vi "FPGA_acquisition - 9205.vi"(8 "error in (no error)":errorcluster, 10 "pound in":refnum<class "Pound.lvclass">, 11 "qbus in":refnum<class "Qbus.lvclass">) -> (0 "error out":errorcluster)   [LabVIEW 2015]
uses:
  <vilib>/addons/Qbus/Qbus.lvclass
  <vilib>/NI/Software Watchdog/Pound/Pound.lvclass
  <vilib>/addons/InsightCM/Devices/Shared/AcquireBaseLoop/controls/State.ctl
  <vilib>/addons/InsightCM/Devices/Shared/AcquireBaseLoop/controls/Configuration.ctl
  <vilib>/addons/InsightCM/Devices/Shared/AcquireBaseLoop/controls/TachometerConfig.ctl
  <vilib>/addons/InsightCM/Devices/Shared/AcquireBaseLoop/controls/FixedSizeArrays.ctl
  <vilib>/LabVIEW Targets/FPGA/cRIO/shared/nicrio_ModuleControls/nicrio_cRIO-9232_ConfigModeRing.ctl
  <vilib>/addons/InsightCM/Devices/Shared/cRIOWfmAcq/subVIs/RIO Wfm Cust Ctrls/rwfm_SamplingInfo.ctl
  <vilib>/addons/InsightCM/Devices/Shared/AcquireBaseLoop/controls/Group.ctl
  <vilib>/addons/InsightCM/Devices/Shared/AcquireBaseLoop/controls/Channel.ctl
  <vilib>/addons/InsightCM/Utilities/ChannelStatus/controls/RangeParams.ctl
  <vilib>/addons/InsightCM/Devices/Shared/AcquireBaseLoop/FpgaAcquisition923x.lvlib
  <vilib>/addons/InsightCM/Devices/Shared/TdmsCreator/TdmsCreator.lvlib
  <vilib>/addons/InsightCM/Devices/Shared/TagPublish/TagPublish.lvlib
  <vilib>/addons/InsightCM/Devices/Shared/FPGABitfileManager/FPGABitfileManager.lvlib
  <vilib>/addons/InsightCM/Devices/Shared/cRIOWfmAcq/cRIOWfmLib.lvlib
  <vilib>/addons/InsightCM/Devices/Shared/DataFlow/DataFlow.lvlib
  <vilib>/addons/InsightCM/Devices/Shared/QbusHelpers/QbusHelper.lvlib
  <vilib>/NI/Software Watchdog/Watchdog/Watchdog.lvclass
  <vilib>/addons/InsightCM/Utilities/ChannelStatus/ChannelStatus.lvlib
panel:
  in  "Waveform Groups Empty?":bool
  out "Numeric":i32
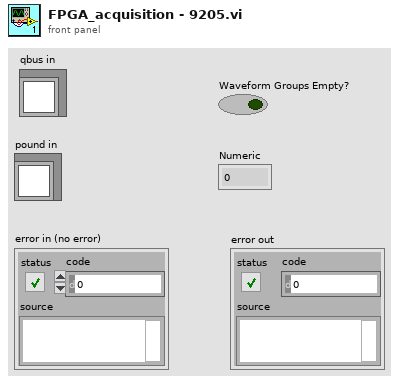
[diagram p1: front panel]
types:
  T1 = typedef "FpgaAcquisition923x.lvlib/Configuration.ctl" = cluster{"NumberOfModules":i16, "Dynamic FPGA VI Ref":refnum<k20>, "KeyphasorX3":T2[], "FixedSizeX24":T3, "SamplingInfo":T5, "BlockSize (sec)":dbl, "Samples To Read (per chan)":i32, "RunningAcquisitionLength":dbl, "Settling Time":dbl, "Waveform Groups":T6[], "Acquisition Block Number":i32, "Device Name":string, "ValidConfig":bool}
  T2 = typedef "FpgaAcquisition923x.lvlib/TachometerConfig.ctl" = cluster{"slope":enum16{"falling", "rising"}, "threshold":dbl, "hysteresis":dbl}
  T3 = typedef "FpgaAcquisition923x.lvlib/FixedSizeArrays.ctl" = cluster{"EnabledChannels":bool[], "Sensitivity":dbl[], "InputConfig":T4[]}
  T4 = typedef "nicrio_cRIO-9232_ConfigModeRing.ctl" = u8
  T5 = typedef "cRIOWfmLib.lvlib/rwfm_SamplingInfo.ctl" = cluster{"Number of Channels":i32, "Sampling Rate":dbl, "Channels":string[], "Units":string[]}
  T6 = typedef "FpgaAcquisition923x.lvlib/Group.ctl" = cluster{"Name":string, "Speed Reference":string, "Channels":T7[]}
  T7 = typedef "FpgaAcquisition923x.lvlib/Channel.ctl" = cluster{"Name":string, "Status Tag":string, "RangeCheck":T8}
  T8 = typedef "ChannelStatus.lvlib/RangeParams.ctl" = cluster{"Enabled":bool, "Max":dbl, "Min":dbl}
  T9 = typedef "FpgaAcquisition923x.lvlib/State.ctl" = enum16{"Unconfigured", "Configured"}
  T10 = typedef "TagPublish.lvlib/PointToPublish.ctl" = cluster{"Id":string, "datatype":T11}
  T11 = typedef "PointValueMap.lvlib/DataTypes.ctl" = enum16{"single", "double", "i32", "string", "variant"}
  T12 = typedef "TdmsCreator.lvlib/RegisterWaveformTdmsPropertiesRoutedMessage.ctl" = cluster{"DataGroup":string, "TdmsGroup":string, "Channels":T13[]}
  T13 = typedef "TdmsCreator.lvlib/Waveform.ctl" = cluster{"ChannelName":string, "Properties":variant, "Write Wfm":bool}
  T14 = typedef "DataFlow.lvlib/Data.ctl" = cluster{"DataGroup":string, "Waveforms":T15, "Map":T16}
  T15 = typedef "wfmSGL_DVR.ctl" = refnum<data-value>
  T16 = typedef "PointValueMap.lvlib/PointMap.ctl" = refnum<data-value>
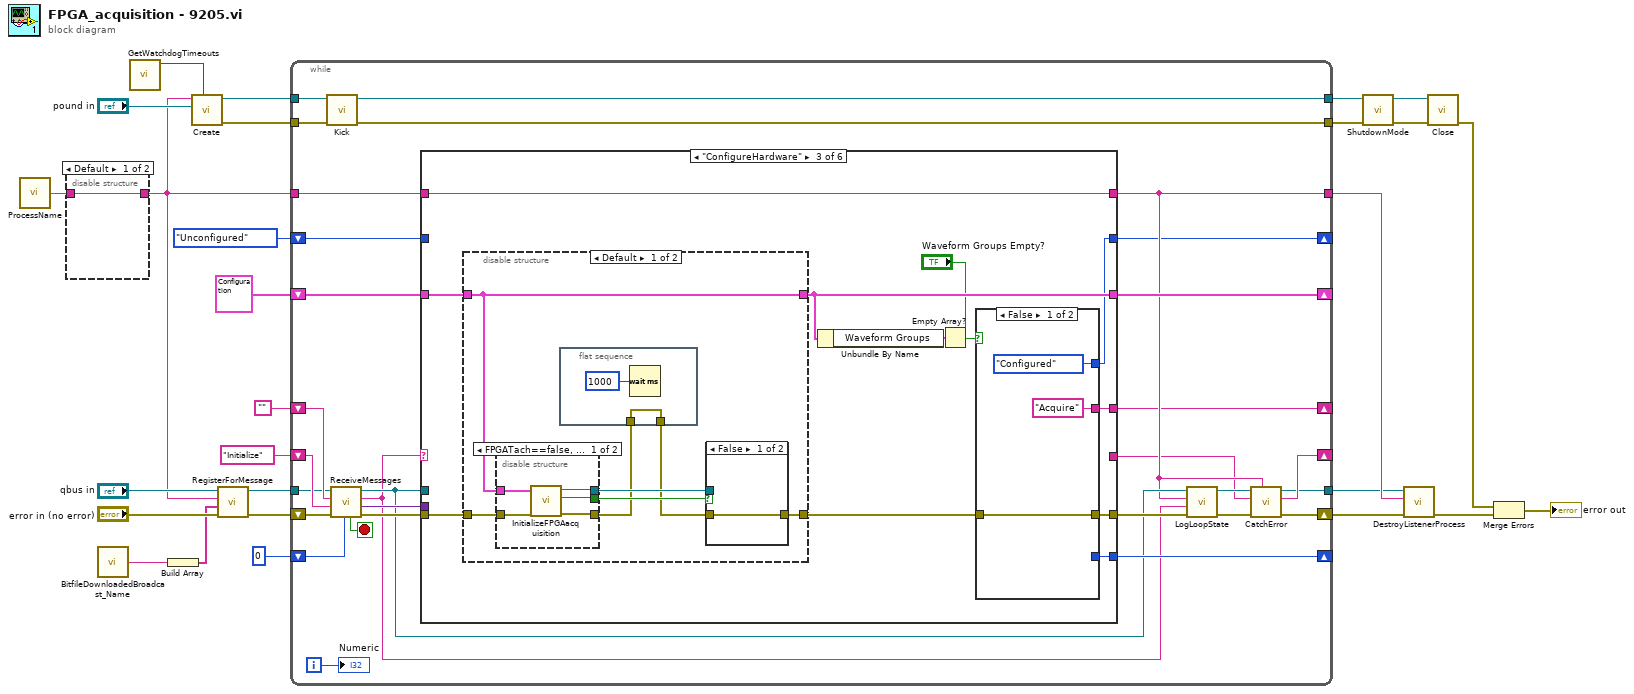
[diagram p0: block diagram]
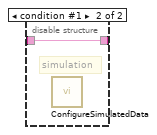
[diagram p2: hidden frame]
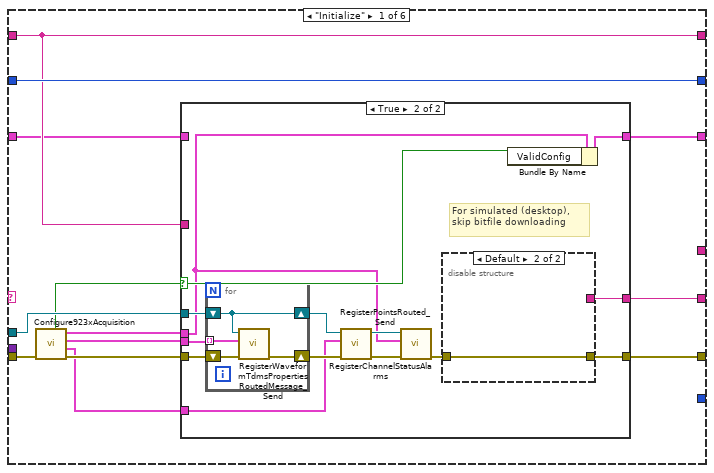
[diagram p3: hidden frame]
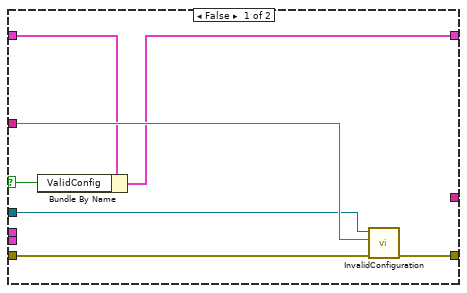
[diagram p4: hidden frame]
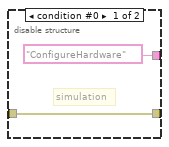
[diagram p5: hidden frame]
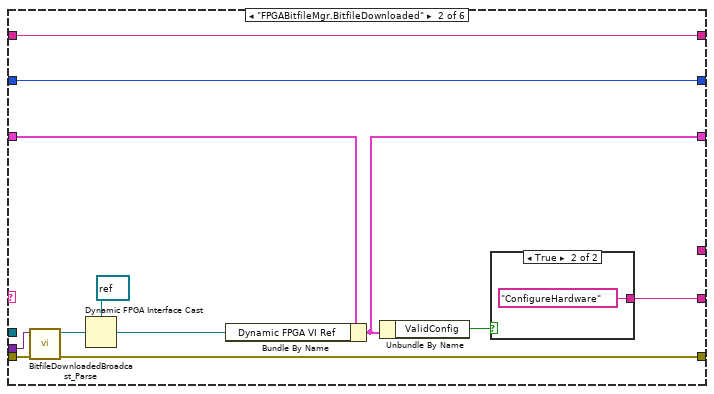
[diagram p6: hidden frame]
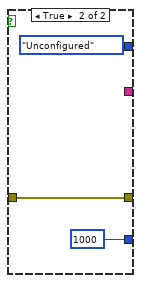
[diagram p8: hidden frame]
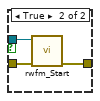
[diagram p9: hidden frame]
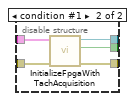
[diagram p10: hidden frame]
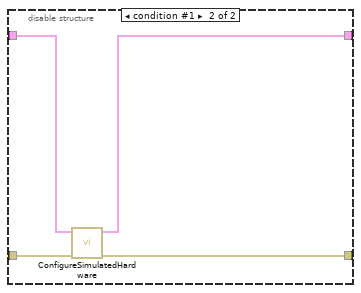
[diagram p11: hidden frame]
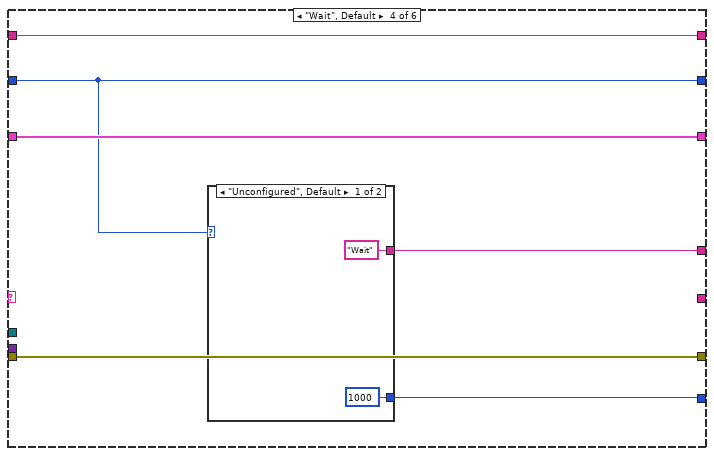
[diagram p12: hidden frame]
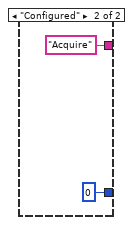
[diagram p13: hidden frame]
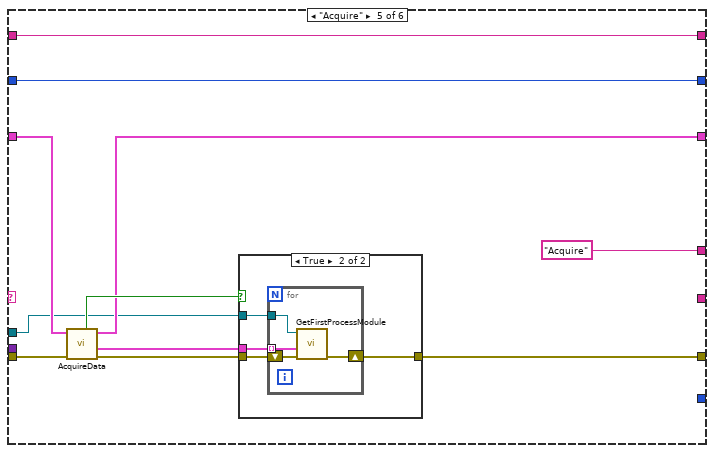
[diagram p14: hidden frame]
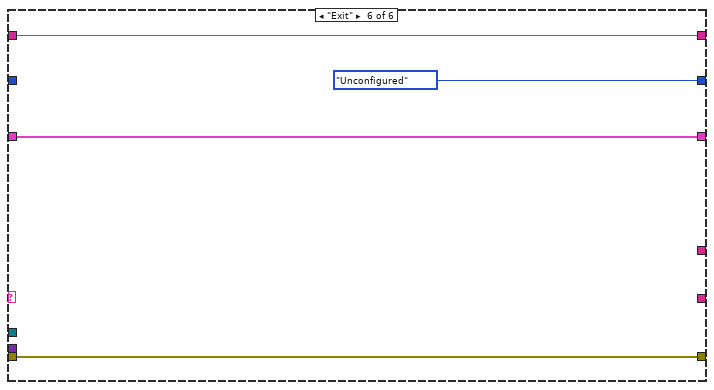
[diagram p16: hidden frame]
diagram:
  n1 = call <vilib>:"ProcessName.vi"() -> ("process name"=w5:string)  [unwired: 5 in]
  n2 = disable-structure shown="Default" {
    disable-tunnel: [w28 w29] -> w6
    disable-tunnel: w5 -> [w28 w29]
    frame condition #0 (active) {
    }
    frame condition #1 {
      # "simulation"
      n3 = call <vilib>:"ConfigureSimulatedData.vi"() -> ()  [unwired: 11 in, 1 out]
    }
  }
  n4 = call <vilib>:"BitfileDownloadedBroadcast_Name.vi"() -> ("message name"=w8:string)  [unwired: 5 in]
  n5 = call <vilib>:"GetWatchdogTimeouts.vi"() -> ("software timeout"=w1:u32)  [unwired: 10 in, 1 out]
  n6 = Build Array(w8) -> (w9:string[])
  n7 = call <vilib>:"Create.vi"("Execution Timeout (ms)"=w1, "Pound"="pound in", "Name"=w6) -> ("error out"=w22:errorcluster, "Watchdog"=w23:refnum<data-value>)  [unwired: 7 in]
  n8 = call <vilib>:"RegisterForMessage.vi"("error in (no error)"="error in (no error)", "message names"=w9, "process name"=w6, "Qbus in"="qbus in") -> ("error in (no error)"=w11:errorcluster, "Qbus out"=w12:refnum<class "Qbus.lvclass">)  [unwired: 6 in]
  n9 = while {
    shift-right: [w46] -> w2
    shift-left: w11 -> [w53]
    shift-right: [w36] -> _
    shift-left: "" -> [w55]
    shift-right: [w59] -> _
    shift-left: T1 {"NumberOfModules"=0, "Dynamic FPGA VI Ref"=refnum, "KeyphasorX3"=[], "FixedSizeX24"={"EnabledChannels"=[], "Sensitivity"=[], "InputConfig"=[]}, "SamplingInfo"={"Number of Channels"=4, "Sampling Rate"=4.0, "Channels"=[], "Units"=[]}, "BlockSize (sec)"=0.0, "Samples To Read (per chan)"=0, "RunningAcquisitionLength"=0.0, "Settling Time"=0.0, "Waveform Groups"=[], "Acquisition Block Number"=0, "Device Name"="", "ValidConfig"=FALSE} ("Config out") -> [w58]
    shift-right: [w34] -> _
    shift-left: State."Unconfigured" ("loop state") -> [w57]
    shift-right: [w56] -> _
    shift-left: 0 ("milliseconds to wait") -> [w51]
    shift-right: [w44] -> _
    shift-left: "Initialize" -> [w54]
    tunnel: w12 -> [w52]
    tunnel: w6 -> [w31]
    tunnel: [w42] -> w3
    tunnel: [w37] -> w25
    tunnel: w23 -> [w41]
    tunnel: w22 -> [w40]
    tunnel: [w39] -> w19
    tunnel: [w38] -> w18
    i -> [w30]
    stop <- w32 stop-if-true
    n10 = call <vilib>:"Kick.vi"("error in (no error)"=w40, "Watchdog"=w41) -> ("error out"=w38:errorcluster, "Watchdog"=w39:refnum<data-value>)  [unwired: 8 in]
    n11 = call <vilib>:"ReceiveMessages.vi"("timeout(100)"=w51, "error in (no error)"=w53, "priority action"=w54, "default action"=w55, "qbus in"=w52) -> ("error out"=w50:errorcluster, "msg value"=w49:variant, "action"=w33:string, "qbus out"=w45:refnum<class "Qbus.lvclass">, "exit"=w32:bool)  [unwired: 2 in]
    n12 = case shown="\"ConfigureHardware\"" w33 {
      tunnel: w50 -> [w70 w104 w122 w163 w170 w188]
      tunnel: [w65 w103 w117 w163 w169 w188] -> w47
      tunnel: [_ _ w124 w161 "Acquire" _] -> w36
      tunnel: [w60 w102 w119 w162 w173 w191] -> w59
      tunnel: w58 -> [w61 w111 w123 w162 w174 w191]
      tunnel: w57 -> [w67 w107 _ w158 w172 _]
      tunnel: [_ _ w116 w159 _ _] -> w56
      tunnel: w31 -> [w63 w112 w121 w160 w171 w189]
      tunnel: w49 -> [_ w105 _ _ _ _]
      tunnel: w45 -> [w69 _ _ _ w168 _]
      tunnel: [w63 w112 w121 w160 w171 w189] -> w37
      tunnel: [w68 w108 _ _ _ _] -> w35
      tunnel: [w67 w107 w115 w158 w172 State."Unconfigured" ("loop state")] -> w34
      frame "Initialize" {
        n13 = call <vilib>:"Configure923xAcquisition.vi"("error in (no error)"=w70) -> ("error out"=w72:errorcluster, "Register Channel Status Tags"=w66:T10[], "Register Waveform TDMS Properties"=w71:T12[], "923x Acquisition Config"=w64:T1, "valid"=w62:bool)  [unwired: 6 in]
        n14 = case shown="True" w62 {
          selector: w62 -> [w75 w81]
          tunnel: w72 -> [w73 w93]
          tunnel: w71 -> [_ w92]
          tunnel: w69 -> [w74 w91]
          tunnel: [_ w90] -> w68
          tunnel: w66 -> [_ w88]
          tunnel: [w79 w83] -> w65
          tunnel: w64 -> [_ w80]
          tunnel: w63 -> [w78 _]
          tunnel: w61 -> [w77 _]
          tunnel: [w76 w82] -> w60
          frame False {
            n15 = Bundle By Name(cluster=w77, "ValidConfig"=w75) -> (w76:T1)
            n16 = call <vilib>:"InvalidConfiguration.vi"("error in (no error)"=w73, "description"=w78, "Qbus in"=w74) -> ("error out"=w79:errorcluster)  [unwired: 7 in, 1 out]
          }
          frame True {
            # "For simulated (desktop),\nskip bitfile downloading"
            n17 = for {
              shift-right: [w99] -> w89
              shift-left: w93 -> [w100]
              tunnel: w92 -> [w98] mode=indexing
              shift-right: [w97] -> w87
              shift-left: w91 -> [w97]
              n18 = call <vilib>:"RegisterWaveformTdmsPropertiesRoutedMessage_Send.vi"("error in (no error)"=w100, "register waveform"=w98, "Qbus in"=w97) -> ("error out"=w99:errorcluster)  [unwired: 7 in, 1 out]
            }
            n19 = call <vilib>:"RegisterPointsRouted_Send.vi"("error in (no error)"=w89, "points"=w88, "Qbus in"=w87) -> ("error out"=w86:errorcluster, "Qbus out"=w84:refnum<class "Qbus.lvclass">)  [unwired: 7 in]
            n20 = call <vilib>:"RegisterChannelStatusAlarms.vi"("error in (no error)"=w86, "923x Acquisition Config"=w80, "Qbus in"=w84) -> ("error out"=w85:errorcluster)  [unwired: 8 in]
            n21 = disable-structure shown="Default" {
              disable-tunnel: w85 -> [w94 w96]
              disable-tunnel: [w94 w96] -> w83
              disable-tunnel: ["ConfigureHardware" _] -> w90
              frame condition #0 {
                # "simulation"
              }
              frame condition #1 (active) {
              }
            }
            n22 = Bundle By Name(cluster=w80, "ValidConfig"=w81) -> (w82:T1)
          }
        }
      }
      frame "FPGABitfileMgr.BitfileDownloaded" {
        n23 = call <vilib>:"BitfileDownloadedBroadcast_Parse.vi"("error in (no error)"=w104, "data"=w105) -> ("error out"=w103:errorcluster, "FPGA reference"=w106:refnum<k20>)  [unwired: 8 in]
        n24 = Dynamic FPGA Interface Cast(Session In=refnum<k20> refnum ("Dynamic FPGA VI Ref"), Type=w106) -> (Session Out=w110:refnum<k20>)
        n25 = Bundle By Name(cluster=w111, "Dynamic FPGA VI Ref"=w110) -> (w102:T1)
        n26 = Unbundle By Name(w102) -> ("ValidConfig"=w101:bool)
        n27 = case shown="True" w101 {
          tunnel: [_ "ConfigureHardware"] -> w108
          frame False {
          }
          frame True {
          }
        }
      }
      frame "ConfigureHardware" {
        n28 = disable-structure shown="Default" {
          disable-tunnel: w123 -> [w134 w155]
          disable-tunnel: w122 -> [w137 w157]
          disable-tunnel: [w136 w156] -> w118
          disable-tunnel: [w134 w154] -> w119
          frame condition #0 (active) {
            n29 = disable-structure shown="FPGATach==false, Default" {
              disable-tunnel: w137 -> [w147 w153]
              disable-tunnel: [w144 w151] -> w132
              disable-tunnel: w134 -> [w148 w152]
              disable-tunnel: [w146 w150] -> w135
              disable-tunnel: [w145 w149] -> w133
              frame condition #0 (active) {
                n30 = call "InitializeFPGAacquisition.vi"("error in (no error)"=w147, "923x Acquisition Config"=w148) -> ("error out"=w144:errorcluster, "start acquisition?"=w145:bool, "dynamic FPGA VI reference"=w146:refnum<k20>)  [unwired: 5 in, 2 out]
              }
              frame condition #1 {
                n31 = call <vilib>:"InitializeFpgaWithTachAcquisition.vi"("error in (no error)"=w153, "923x Acquisition Config"=w152) -> ("error out"=w151:errorcluster, "start acquisition?"=w149:bool, "dynamic FPGA VI reference"=w150:refnum<k20>)  [unwired: 7 in]
              }
            }
            n32 = flat-sequence {
              tunnel: [w138] -> w131
              tunnel: w132 -> [w138]
              frame #0 {
                n33 = Wait (ms)(milliseconds to wait=u32 1000) -> ()  [unwired: 1 out]
              }
            }
            n34 = case shown="False" w133 {
              tunnel: [w140 w143] -> w136
              tunnel: w131 -> [w140 w142]
              tunnel: w135 -> [_ w141]
              frame False {
              }
              frame True {
                n35 = call <vilib>:"rwfm_Start.vi"("error in"=w142, "Dynamic FPGA VI Reference"=w141) -> ("error out"=w143:errorcluster)  [unwired: 7 in, 2 out]
              }
            }
          }
          frame condition #1 {
            n36 = call <vilib>:"ConfigureSimulatedHardware.vi"("error in (no error)"=w157, "configuration"=w155) -> ("error out"=w156:errorcluster, "configuration out"=w154:T1)  [unwired: 8 in]
          }
        }
        n37 = Unbundle By Name(w119) -> ("Waveform Groups"=w120:T6[])
        n38 = Empty Array?(array=w120) -> ()  [unwired: 1 out]
        n39 = case shown="False" "Waveform Groups Empty?" {
          tunnel: ["Acquire" _] -> w124
          tunnel: [w126 w130] -> w117
          tunnel: w118 -> [w126 w130]
          tunnel: [_ 1000] -> w116
          tunnel: [State."Configured" ("loop state") State."Unconfigured" ("loop state")] -> w115
          frame False {
          }
          frame True {
          }
        }
      }
      frame "Wait", Default {
        n40 = case shown="\"Unconfigured\", Default" w158 {
          tunnel: ["Wait" "Acquire"] -> w161
          tunnel: [1000 0] -> w159
          frame "Unconfigured", Default {
          }
          frame "Configured" {
          }
        }
      }
      frame "Acquire" {
        n41 = call <vilib>:"AcquireData.vi"("error in (no error)"=w170, "923x acquisition config"=w174) -> ("error out"=w177:errorcluster, "dataflow messages"=w176:T14[], "923x acquisition config out"=w173:T1, "settling time requirement met?"=w175:bool)  [unwired: 6 in]
        n42 = case shown="True" w175 {
          tunnel: w177 -> [w179 w181]
          tunnel: [w179 w180] -> w169
          tunnel: w176 -> [_ w183]
          tunnel: w168 -> [_ w182]
          frame False {
          }
          frame True {
            n43 = for {
              tunnel: w183 -> [w184] mode=indexing
              tunnel: w182 -> [w185]
              shift-right: [w186] -> w180
              shift-left: w181 -> [w187]
              n44 = call <vilib>:"GetFirstProcessModule.vi"("error in (no error)"=w187, "data"=w184, "Qbus in"=w185) -> ("error out"=w186:errorcluster)  [unwired: 7 in, 1 out]
            }
          }
        }
      }
      frame "Exit" {
      }
    }
    n45 = call <vilib>:"LogLoopState.vi"("error in (no error)"=w47, "loop action"=w33, "process name"=w37, "Qbus in"=w45) -> ("error out"=w48:errorcluster, "Qbus out"=w43:refnum<class "Qbus.lvclass">)  [unwired: 6 in]
    n46 = call <vilib>:"CatchError.vi"("source"=w37, "error in (no error)"=w48, "next action in"=w35, "Qbus in"=w43) -> ("error out"=w46:errorcluster, "next action out"=w44:string, "Qbus out"=w42:refnum<class "Qbus.lvclass">)  [unwired: 5 in]
    "Numeric" <- w30
  }
  n47 = call <vilib>:"ShutdownMode.vi"("error in (no error)"=w18, "Watchdog"=w19) -> ("error out"=w20:errorcluster, "Watchdog"=w21:refnum<data-value>)  [unwired: 8 in]
  n48 = call <vilib>:"DestroyListenerProcess.vi"("error in (no error)"=w2, "process name"=w25, "Qbus in"=w3) -> ("error in (no error)"=w16:errorcluster)  [unwired: 7 in, 1 out]
  n49 = call <vilib>:"Close.vi"("error in (no error)"=w20, "Watchdog"=w21) -> ("error out"=w15:errorcluster)  [unwired: 9 in]
  n50 = Merge Errors(w15, w16) -> (→"error out":errorcluster)
